vi "Floor_Negative.vi"(10 "Baseline U8":u8, 11 "Input Value":u8) -> (3 "Output Value":u8)   [LabVIEW 2012]
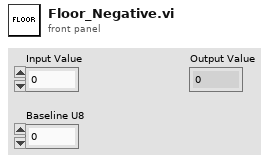
[diagram p1: front panel]
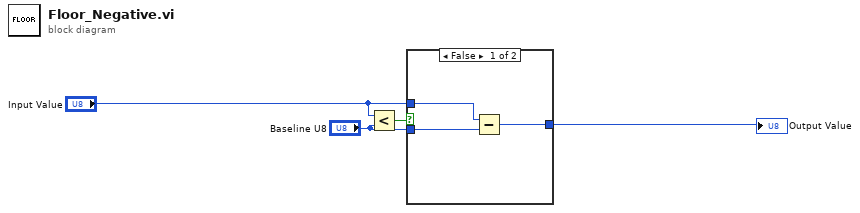
[diagram p0: block diagram]
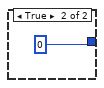
[diagram p2: hidden frame]
diagram:
  n1 = Less?(x="Input Value", y="Baseline U8") -> (x < y?=w3:bool)
  n2 = case shown="False" w3 {
    tunnel: "Input Value" -> [w7 _]
    tunnel: "Baseline U8" -> [w6 _]
    tunnel: [w5 u8 0] -> w4
    frame False {
      n3 = Subtract(x=w7, y=w6) -> (x-y=w5:u8)
    }
    frame True {
    }
  }
  "Output Value" <- w4
